vi "Arm Testing.vi"() -> ()   [LabVIEW 2015]
uses:
  <vilib>/Rock Robotics/WPI/Utilities/WPI_GetSetVariantRefNum.vi
  Robot Global Data.vi
  <vilib>/Utility/inputDevices.llb/keyboardAcquire.vi
panel:
  out "XY Graph":cluster{"X":dbl, "Y":dbl}[](graph)
  in  "Gravity cancelling":dbl(slide) scale=0.0..1.0
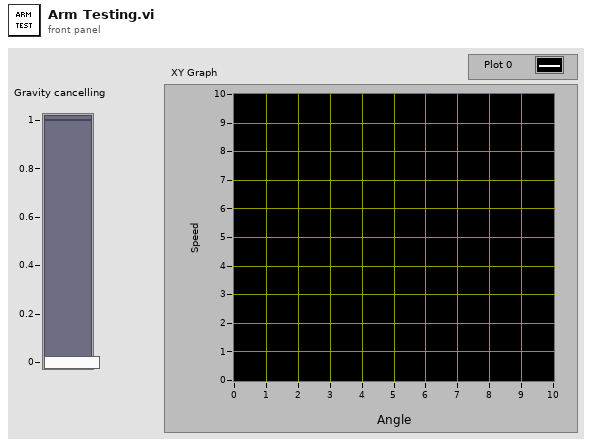
[diagram p1: front panel]
types:
  T1 = typedef "WPI_RobotDriveDevRef.ctl" = cluster{"DevStatus":errorcluster, "Motors[]":T2[], "Square Inputs":bool, "Max Output":dbl}
  T2 = typedef "WPI_MotorControlDeviceRef.ctl" = cluster{"DeviceStatus":errorcluster, "Type":T3, "PWM":cluster{"PWM Channel":T4, "DeadBand":T5}, "CAN":cluster{"Device Number":u8, "Control Mode":T6, "Semaphore":T7, "Max Vout":dbl, "TalonSRX Control Mode":T8}, "Invert":bool}
  T3 = typedef "WPI_MotorControlType.ctl" = enum16{"PWM", "CAN", "CANTalonSRX"}
  T4 = typedef "FPGA_DIOPWMChannel.ctl" = enum8{"PWM 0", "PWM 1", "PWM 2", "PWM 3", "PWM 4", "PWM 5", "PWM 6", "PWM 7", "PWM 8", "PWM 9", "PWM MXP 0", "PWM MXP 1", "PWM MXP 2", "PWM MXP 3", "PWM MXP 4", "PWM MXP 5", "PWM MXP 6", "PWM MXP 7", "PWM MXP 8", "PWM MXP 9", "Invalid"}
  T5 = typedef "WPI_PWMDeadband.ctl" = cluster{"Name":string, "maxPositivePwm":i32, "minPositivePwm":i32, "centerPwm":i32, "maxNegativePwm":i32, "minNegativePwm":i32, "angularRange":u16}
  T6 = typedef "WPI_CANJaguar_ControlMode.ctl" = enum8{"Percent VBus", "Current", "Speed", "Position", "Voltage"}
  T7 = typedef "Semaphore RefNum" = refnum<k1>
  T8 = typedef "WPI_CANTalonSRX_APIControlMode.ctl" = enum8{"Percent VBus", "Speed", "Position", "Slave", "Unchanged / Invalid", "Voltage Compensation", "Current", "Motion Profile"}
  T9 = enum16{"0", "1", "2", "3", "4", "5", "6", "7", "8", "9", "A", "B", "C", "D", "E", "F", "G", "H", "I", "J", "K", "L", "M", "N", "O", "P", "Q", "R", "S", "T", "U", "V", "W", "X", "Y", "Z", "F1", "F2", "F3", "F4", "F5", "F6", "F7", "F8", "F9", "F10", "F11", "F12", "F13", "F14", "F15", "ADD", "BACK", "BACKSLASH", "CAPITAL", "COMMA", "DECIMAL", "DELETE", "DIVIDE", "DOWN", "END", "EQUALS", "ESCAPE", "GRAVE (`)", "HOME", "INSERT", "LBRACKET", "LCONTROL", "LEFT", "L ALT", "LSHIFT", "LWIN", "MINUS", "MULTIPLY", "NEXT", "NUMLOCK", "NUMPAD_0", "NUMPAD_1", "NUMPAD_2", "NUMPAD_3", "NUMPAD_4", "NUMPAD_5", "NUMPAD_6", "NUMPAD_7", "NUMPAD_8", "NUMPAD_9", "PAUSE", "PERIOD", "PRIOR (PG UP)", "RBRACKET", "RCONTROL", "RETURN", "RIGHT", "R ALT", "RSHIFT", "RWIN", "SCROLL", "SEMICOLON", "SLASH", "SPACE", "SUBTRACT", "TAB", "UP", "ENTER (num pad)", "' (quote)"}
  T10 = enum16{"0", "1", "2", "3", "4", "5", "6", "7", "8", "9", "A", "B", "C", "D", "E", "F", "G", "H", "I", "J", "K", "L", "M", "N", "O", "P", "Q", "R", "S", "T", "U", "V", "W", "X", "Y", "Z", "F1", "F2", "F3", "F4", "F5", "F6", "F7", "F8", "F9", "F10", "F11", "F12", "F13", "F14", "F15", "ADD", "BACK", "BACKSLASH", "CAPITAL", "COMMA", "DECIMAL", "DELETE", "DIVIDE", "DOWN", "END", "EQUALS", "ESCAPE", "GRAVE (`)", "HOME", "INSERT", "LBRACKET", "LCONTROL", "LEFT", "L ALT", "LSHIFT", "LWIN", "MINUS", "MULTIPLY", "NEXT", "NUMLOCK", "NUMPAD_0", "NUMPAD_1", "NUMPAD_2", "NUMPAD_3", "NUMPAD_4", "NUMPAD_5", "NUMPAD_6", "NUMPAD_7", "NUMPAD_8", "NUMPAD_9", "PAUSE", "PERIOD", "PRIOR (PG UP)", "RBRACKET", "RCONTROL", "RETURN", "RIGHT", "R ALT", "RSHIFT", "RWIN", "SCROLL", "SEMICOLON", "SLASH", "SPACE", "SUBTRACT", "TAB", "UP", "ENTER (num pad)", "' (quote)"}[]
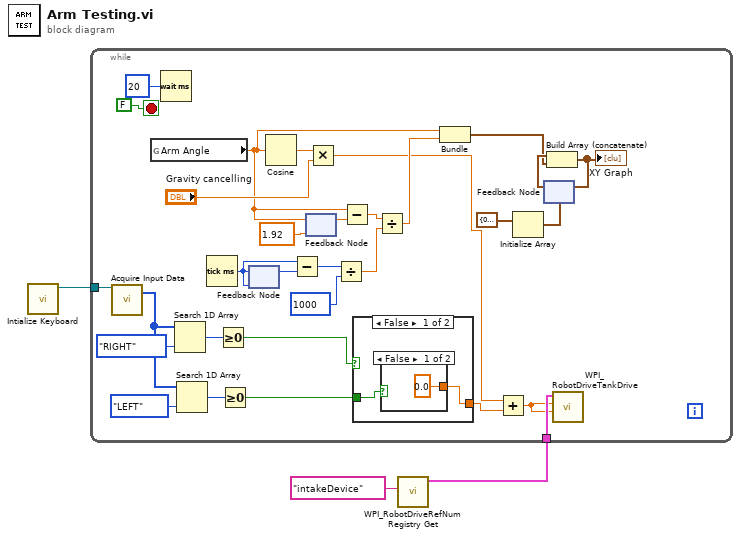
[diagram p0: block diagram]
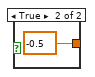
[diagram p2: hidden frame]
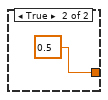
[diagram p3: hidden frame]
diagram:
  n1 = call <vilib>:"Intialize Keyboard.vi"() -> ("device ID"=w1:refnum<k1>)  [unwired: 10 in, 1 out]
  n2 = call <vilib>:"WPI_RobotDriveRefNum Registry Get.vi"("refnum name"="intakeDevice") -> ("RobotDriveDevRef"=w2:T1)  [unwired: 9 in, 1 out]
  n3 = while {
    tunnel: w2 -> [w15]
    tunnel: w1 -> [w14]
    stop <- FALSE stop-if-true
    n4 = call-poly <vilib>:"Acquire Input Data.vi"("device ID"=w14) -> ("keys pressed"=w8:T10)  [unwired: 16 in, 2 out]
    n5 = global read "Robot Global Data.vi" "Arm Angle"() -> (w22:dbl)
    n6 = Wait (ms)(milliseconds to wait=u32 20) -> ()  [unwired: 1 out]
    n7 = Search 1D Array(1D array=w8, element=T9."RIGHT") -> (index of element=w12:i32)  [unwired: 1 in]
    n8 = Search 1D Array(1D array=w8, element=T9."LEFT") -> (index of element=w10:i32)  [unwired: 1 in]
    n9 = Tick Count (ms)() -> (millisecond timer value=w28:u32)
    n10 = Greater Or Equal To 0?(x=w12) -> (x >= 0?=w11:bool)
    n11 = Greater Or Equal To 0?(x=w10) -> (x >= 0?=w7:bool)
    n12 = feedback #1(w28) -> (w27:u32)
    n13 = feedback-in #1(w28) -> ()
    n14 = Cosine(x=w22) -> (cos(x)=w34:dbl)
    n15 = Subtract(x=w28, y=w27) -> (x-y=w26:u32)
    n16 = feedback #2(1.92 ("Arm Angle")) -> (w29:dbl)
    n17 = feedback-in #2(w22) -> ()
    n18 = Multiply(x=w34, y="Gravity cancelling") -> (x*y=w4:dbl)
    n19 = Divide(x=w26, y=u32 1000) -> (x/y=w23:dbl)
    n20 = Subtract(x=w22, y=w29) -> (x-y=w24:dbl)
    n21 = case shown="False" w11 {
      tunnel: w7 -> [w36 _]
      tunnel: [w35 0.5 ("Arm Angle")] -> w6
      frame False {
        n22 = case shown="False" w36 {
          tunnel: [0.0 ("Arm Angle") -0.5 ("Arm Angle")] -> w35
          frame False {
          }
          frame True {
          }
        }
      }
      frame True {
      }
    }
    n23 = Divide(x=w24, y=w23) -> (x/y=w21:dbl)
    n24 = Bundle("Arm Angle"=w22, w21) -> (w17:cluster{"Arm Angle":dbl, dbl})  [unwired: 1 in]
    n25 = Add(x=w4, y=w6) -> (x+y=w5:dbl)
    n26 = Initialize Array(cluster{"Arm Angle":dbl, dbl} {"Arm Angle"=0.0, 0.0} ("output cluster")) -> (w19:cluster{"Arm Angle":dbl, dbl}[])  [unwired: 1 in]
    n27 = feedback #3(w19) -> (w18:cluster{"Arm Angle":dbl, dbl}[])
    n28 = Build Array (concatenate)(w18, w17) -> (w16:cluster{"Arm Angle":dbl, dbl}[])
    "XY Graph" <- w16
    n29 = feedback-in #3(w16) -> ()
    n30 = call <vilib>:"WPI_RobotDriveTankDrive.vi"("Right axis value"=w5, "Left axis value"=w5, "RobotDriveDevRef"=w15) -> ()  [unwired: 6 in, 3 out]
  }
